vi "var_global.vi"(3 "Param in":T2={"Play"=FALSE, "num of sampl"=0, "sound format"={"sample rate (S/s)"=22050.0, "number of channels"=2, "bits per sample"=16}}, 6 "Action":enum16{"Set", "Get"}(ring)) -> (11 "Param out":T2={"Play"=FALSE, "num of sampl"=0, "sound format"={"sample rate (S/s)"=22050.0, "number of channels"=2, "bits per sample"=16}})   [LabVIEW 2018]
uses:
  <vilib>/sound2/lvsound2.llb/Sound Data Format.ctl
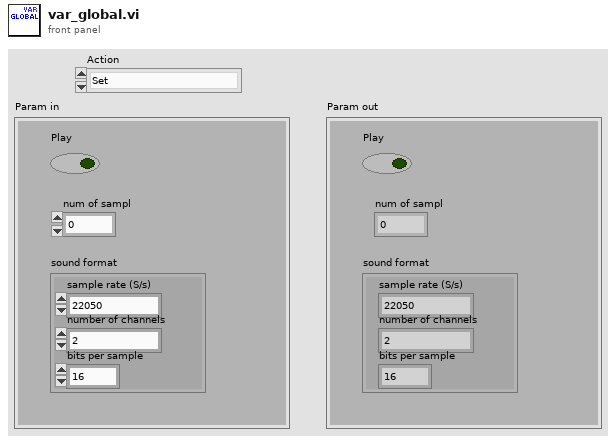
[diagram p1: front panel]
types:
  T1 = typedef "Sound Data Format.ctl" = cluster{"sample rate (S/s)":dbl, "number of channels":i32, "bits per sample":i32}
  T2 = cluster{"Play":bool, "num of sampl":i32, "sound format":T1}
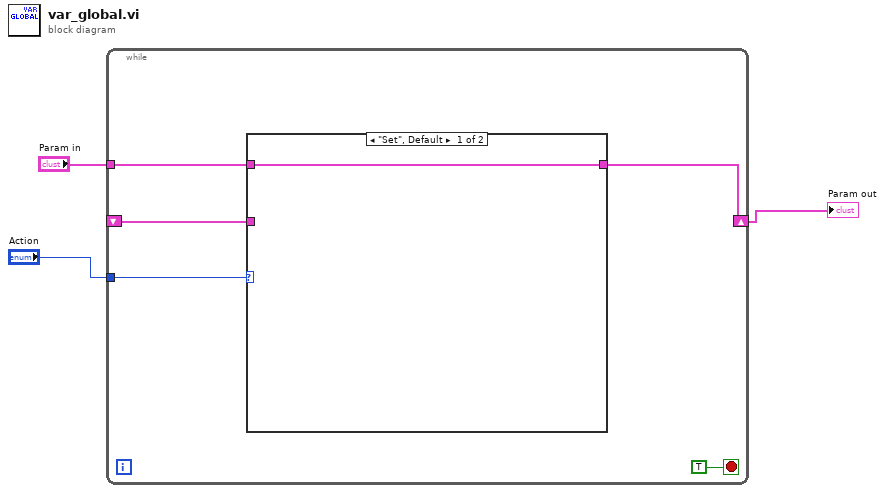
[diagram p0: block diagram]
diagram:
  n1 = while {
    tunnel: "Action" -> [w8]
    shift-right: [w6] -> w1
    shift-left: _ -> [w5]
    tunnel: "Param in" -> [w7]
    stop <- TRUE stop-if-true
    n2 = case shown="\"Set\", Default" w8 {
      tunnel: w7 -> [w9 _]
      tunnel: [w9 w10] -> w6
      tunnel: w5 -> [_ w10]
      frame "Set", Default {
      }
      frame "Get" {
      }
    }
  }
  "Param out" <- w1
